vi "RubikTurnFSM2.vi"(1 "Turn":T3=enum."ccw", 2 "Servo Enum":T1) -> (0 "Turn State (out)":T2)   [LabVIEW 2017]
uses:
  Projekt-RubikLibrary/ServoCCWControl.ctl
  Projekt-RubikLibrary/ServoAbsAngleControl.ctl
  Projekt-RubikLibrary/ServoEnumControl.ctl
  Projekt-RubikLibrary/RubikLibrary.lvlib
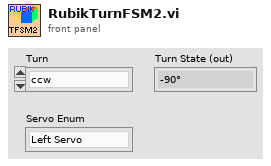
[diagram p1: front panel]
types:
  T1 = typedef "RubikLibrary.lvlib/ServoEnumControl.ctl" = enum16{"Left Servo", "Front Servo", "Right Servo"}
  T2 = typedef "RubikLibrary.lvlib/ServoAbsAngleControl.ctl" = enum16{"-90°", "0°", "+90°"}
  T3 = typedef "RubikLibrary.lvlib/ServoCCWControl.ctl" = enum16{"cw", "ccw"}
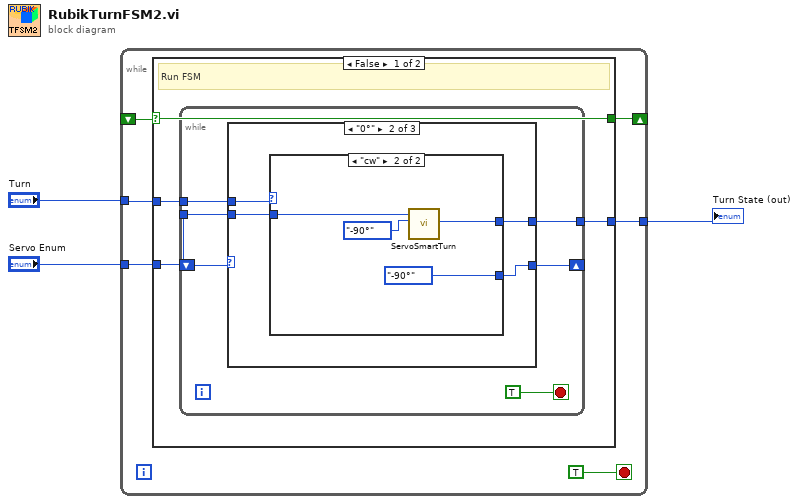
[diagram p0: block diagram]
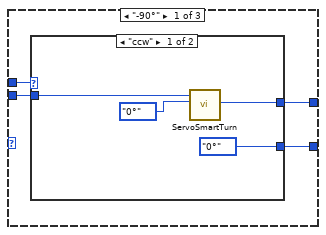
[diagram p2: hidden frame]
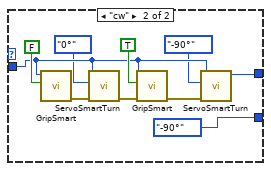
[diagram p3: hidden frame]
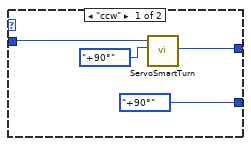
[diagram p4: hidden frame]
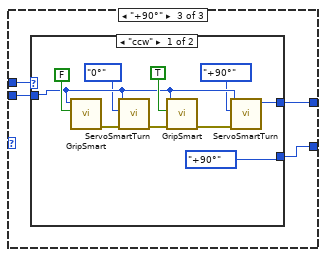
[diagram p5: hidden frame]
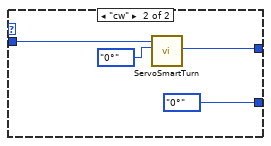
[diagram p6: hidden frame]
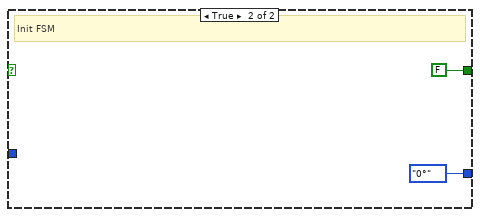
[diagram p7: hidden frame]
diagram:
  n1 = while {
    tunnel: "Turn" -> [w9]
    tunnel: [w8] -> w2
    tunnel: "Servo Enum" -> [w7]
    shift-right: [w4] -> _
    shift-left: _ -> [w5]
    stop <- TRUE stop-if-true
    n2 = case shown="False" w5 {
      selector: w5 -> [w10 _]
      tunnel: w9 -> [w13 _]
      tunnel: [w12 ServoAbsAngleControl."0°" ("Turn State (out)")] -> w8
      tunnel: w7 -> [w11 _]
      tunnel: [w10 FALSE] -> w4
      frame False {
        # "Run FSM"
        n3 = while {
          shift-right: [w18] -> _
          shift-left: _ -> [w19]
          tunnel: w11 -> [w16]
          tunnel: [w15] -> w12
          tunnel: w13 -> [w14]
          stop <- TRUE stop-if-true
          n4 = case shown="\"0°\"" w19 {
            tunnel: [w23 w41 w53] -> w18
            tunnel: w16 -> [w22 w40 w52]
            tunnel: [w21 w39 w51] -> w15
            tunnel: w14 -> [w20 w38 w50]
            frame "-90°" {
              n5 = case shown="\"ccw\"" w20 {
                tunnel: [ServoAbsAngleControl."0°" ("Enum 2") ServoAbsAngleControl."-90°" ("Enum 2")] -> w23
                tunnel: w22 -> [w26 w31]
                tunnel: [w25 w30] -> w21
                frame "ccw" {
                  n6 = call "ServoSmartTurn.vi"("Turn to (in)"=ServoAbsAngleControl."0°" ("Turn to"), "Servo"=w26) -> ("Turn State (out)"=w25:T2)  [unwired: 8 in, 1 out]
                }
                frame "cw" {
                  n7 = call "GripSmart.vi"("Grip closed (in)"=FALSE ("Turn to (in)"), "Servo"=w31) -> ("error out"=w35:errorcluster)  [unwired: 8 in, 1 out]
                  n8 = call "ServoSmartTurn.vi"("error in"=w35, "Turn to (in)"=ServoAbsAngleControl."0°" ("Turn to"), "Servo"=w31) -> ("error out"=w34:errorcluster)  [unwired: 7 in, 1 out]
                  n9 = call "GripSmart.vi"("error in"=w34, "Grip closed (in)"=TRUE ("Turn to (in)"), "Servo"=w31) -> ("error out"=w33:errorcluster)  [unwired: 7 in, 1 out]
                  n10 = call "ServoSmartTurn.vi"("error in"=w33, "Turn to (in)"=ServoAbsAngleControl."-90°" ("Turn to"), "Servo"=w31) -> ("Turn State (out)"=w30:T2)  [unwired: 7 in, 1 out]
                }
              }
            }
            frame "0°" {
              n11 = case shown="\"cw\"" w38 {
                tunnel: [ServoAbsAngleControl."+90°" ("Enum 2") ServoAbsAngleControl."-90°" ("Enum 2")] -> w41
                tunnel: w40 -> [w44 w48]
                tunnel: [w43 w47] -> w39
                frame "ccw" {
                  n12 = call "ServoSmartTurn.vi"("Turn to (in)"=ServoAbsAngleControl."+90°" ("Turn to"), "Servo"=w44) -> ("Turn State (out)"=w43:T2)  [unwired: 8 in, 1 out]
                }
                frame "cw" {
                  n13 = call "ServoSmartTurn.vi"("Turn to (in)"=ServoAbsAngleControl."-90°" ("Turn to"), "Servo"=w48) -> ("Turn State (out)"=w47:T2)  [unwired: 8 in, 1 out]
                }
              }
            }
            frame "+90°" {
              n14 = case shown="\"ccw\"" w50 {
                tunnel: [ServoAbsAngleControl."+90°" ("Enum 2") ServoAbsAngleControl."0°" ("Enum 2")] -> w53
                tunnel: w52 -> [w57 w66]
                tunnel: [w56 w65] -> w51
                frame "ccw" {
                  n15 = call "GripSmart.vi"("Grip closed (in)"=FALSE ("Turn to (in)"), "Servo"=w57) -> ("error out"=w61:errorcluster)  [unwired: 8 in, 1 out]
                  n16 = call "ServoSmartTurn.vi"("error in"=w61, "Turn to (in)"=ServoAbsAngleControl."0°" ("Turn to"), "Servo"=w57) -> ("error out"=w60:errorcluster)  [unwired: 7 in, 1 out]
                  n17 = call "GripSmart.vi"("error in"=w60, "Grip closed (in)"=TRUE ("Turn to (in)"), "Servo"=w57) -> ("error out"=w59:errorcluster)  [unwired: 7 in, 1 out]
                  n18 = call "ServoSmartTurn.vi"("error in"=w59, "Turn to (in)"=ServoAbsAngleControl."+90°" ("Turn to"), "Servo"=w57) -> ("Turn State (out)"=w56:T2)  [unwired: 7 in, 1 out]
                }
                frame "cw" {
                  n19 = call "ServoSmartTurn.vi"("Turn to (in)"=ServoAbsAngleControl."0°" ("Turn to"), "Servo"=w66) -> ("Turn State (out)"=w65:T2)  [unwired: 8 in, 1 out]
                }
              }
            }
          }
        }
      }
      frame True {
        # "Init FSM"
      }
    }
  }
  "Turn State (out)" <- w2
